vi "extract and prune to time range.vi"(7 "prune?":bool=TRUE, 8 "error in (no error)":errorcluster, 9 "t0":dbl, 10 "time range":dbl=-1.0, 11 "time and val queue":refnum<queue>) -> (0 "error out":errorcluster, 2 "graph":cluster{dbl[], dbl[]}, 3 "time and val queue out":refnum<queue>)   [LabVIEW 2017]
uses:
  typedefs/reading1.ctl
panel:
  out "s? t:f":dbl
  out "max index(es)":i32
  out "min index(es)":i32
  out "min value":dbl
  out "max value":dbl
  out "Array":dbl[](array[numeric])
  out "size(s)":i32
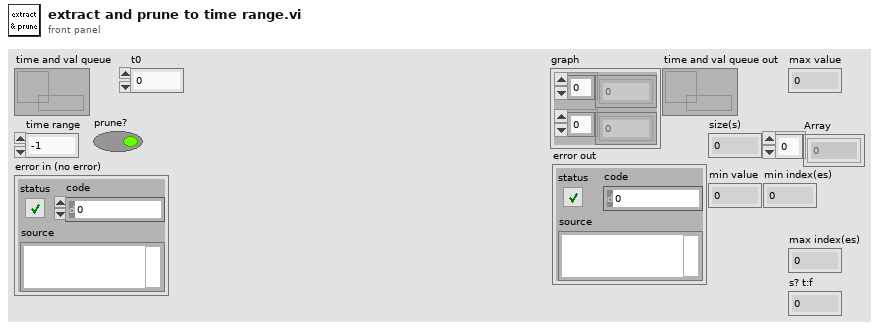
[diagram p1: front panel]
types:
  T1 = typedef "reading1.ctl" = cluster{"time":dbl, "x":dbl, "ms timer":u32}
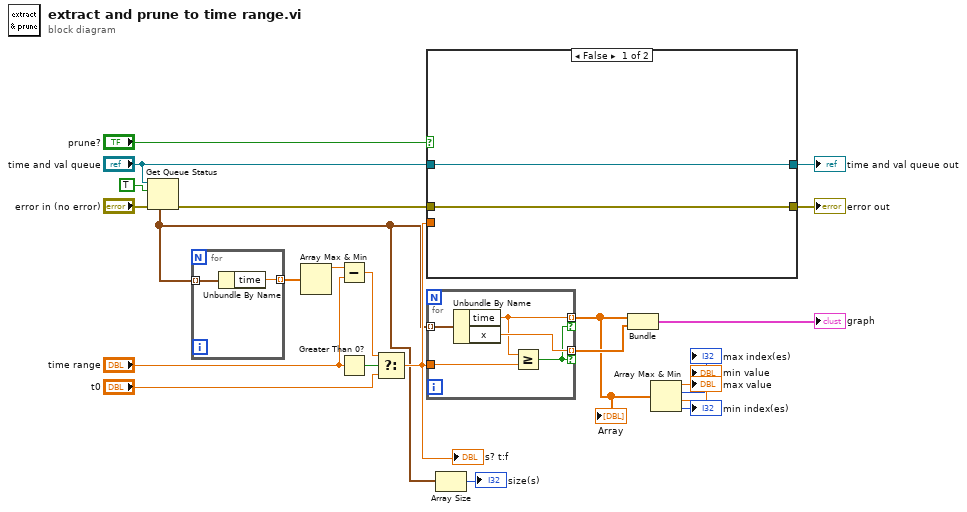
[diagram p0: block diagram]
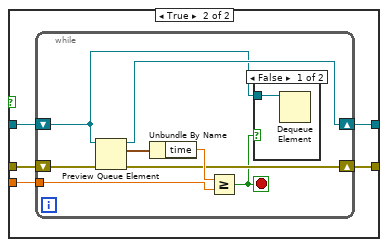
[diagram p2: hidden frame]
diagram:
  n1 = Get Queue Status(queue="time and val queue", return elements? (F)=TRUE, error in (no error)="error in (no error)") -> (error out=w21:errorcluster, elements=w6:T1[])  [unwired: 6 out]
  n2 = for {
    tunnel: w6 -> [w25] mode=indexing
    tunnel: [w24] -> w20 mode=indexing
    n3 = Unbundle By Name(w25) -> ("time"=w24:dbl)
  }
  n4 = Array Max & Min(array=w20) -> (max value=w8:dbl)  [unwired: 3 out]
  n5 = Subtract(x=w8, y="time range") -> (x-y=w18:dbl)
  n6 = Greater Than 0?(x="time range") -> (x > 0?=w19:bool)
  n7 = Select(t=w18, s=w19, f="t0") -> (s? t:f=w10:dbl)
  "s? t:f" <- w10
  n8 = case shown="False" "prune?" {
    tunnel: w21 -> [w27 w32]
    tunnel: [w27 w31] -> w11
    tunnel: [w26 w30] -> w12
    tunnel: "time and val queue" -> [w26 w29]
    tunnel: w10 -> [_ w28]
    frame False {
    }
    frame True {
      n9 = while {
        tunnel: w28 -> [w37]
        shift-right: [w35] -> w31
        shift-left: w32 -> [w40]
        shift-right: [w39] -> w30
        shift-left: w29 -> [w33]
        stop <- w34 stop-if-true
        n10 = Preview Queue Element(queue=w33, error in (no error)=w40) -> (queue out=w39:refnum<queue>, element=w36:T1, error out=w35:errorcluster)  [unwired: 1 in, 1 out]
        n11 = Unbundle By Name(w36) -> ("time"=w38:dbl)
        n12 = Greater Or Equal?(x=w38, y=w37) -> (x >= y?=w34:bool)
        n13 = case shown="False" w34 {
          tunnel: w33 -> [w41 _]
          frame False {
            n14 = Dequeue Element(queue=w41) -> ()  [unwired: 2 in, 4 out]
          }
          frame True {
          }
        }
      }
    }
  }
  "error out" <- w11
  "time and val queue out" <- w12
  n15 = for {
    tunnel: w6 -> [w46] mode=indexing
    tunnel: [w44] -> w7 mode=indexing if=w42
    tunnel: [w45] -> w23 mode=indexing if=w42
    tunnel: w10 -> [w43]
    n16 = Unbundle By Name(w46) -> ("time"=w44:dbl, "x"=w45:dbl)
    n17 = Greater Or Equal?(x=w44, y=w43) -> (x >= y?=w42:bool)
  }
  "Array" <- w7
  n18 = Array Size(array=w6) -> (size(s)=→"size(s)":i32)
  n19 = Bundle(w7, w23) -> (→"graph":cluster{dbl[], dbl[]})  [unwired: 1 in]
  n20 = Array Max & Min(array=w7) -> (max value=→"max value":dbl, max index (indices)=→"max index(es)":i32, min value=→"min value":dbl, min index (indices)=→"min index(es)":i32)
